vi "Reload.vi"(0 "reference in":refnum<class "LcWebView.lvclass">, 5 "Error In":errorcluster) -> (14 "reference out":refnum<class "LcWebView.lvclass">, 19 "Error Out":errorcluster)   [LabVIEW 2020, in "LcWebView.lvclass"]
uses:
  LcWebView.lvclass
  C:/Projects/WebView2/LcWebView/data/Microsoft.Web.WebView2.Core.dll
  data/Microsoft.Web.WebView2.Core.dll
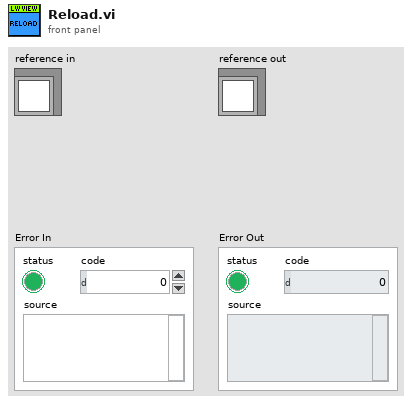
[diagram p1: front panel]
types:
  T1 = typedef "LcWebView.lvclass/ObjectAttributes.ctl" = cluster{"WebView Container":refnum<k24>, "CoreWebViewRef":refnum<k24>, "Status":i32, "Status Message":string, "User Data Folder":path, "DynamicEvents":T2, "BrowserProcessId":u32, "PlotMap":T3, "PlotType":T5}
  T2 = typedef "LcWebView.lvclass/WebViewDynamicEvents.ctl" = cluster{"Event Registration Ref":refnum<event-registration>, "Source event":refnum<user-event>}
  T3 = typedef "LcWebView.lvclass/PlotMap.ctl" = map{string, T4}
  T4 = typedef "LcWebView.lvclass/PlotRef.ctl" = cluster{"PlotType":T5, "PlotTemplate":string}
  T5 = typedef "LcWebView.lvclass/PlotType.ctl" = enum16{"bar", "line", "pie"}
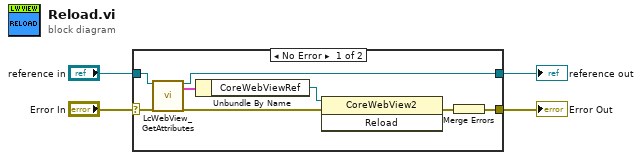
[diagram p0: block diagram]
diagram:
  n1 = case shown="No Error" "Error In" {
    selector: "Error In" -> [w12 w14]
    tunnel: [w9 w14] -> w3
    tunnel: [w10 w13] -> w1
    tunnel: "reference in" -> [w11 w13]
    frame No Error {
      n2 = call "LcWebView_GetAttributes.vi"("reference in"=w11, "error in (no error)"=w12) -> ("reference out"=w10:refnum<class "LcWebView.lvclass">, "Data"=w8:T1, "error out"=w6:errorcluster)  [unwired: 14 in, 1 out]
      n3 = Unbundle By Name(w8) -> ("CoreWebViewRef"=w7:refnum<k24>)
      n4 = invoke class="CoreWebView2" method="Reload"(reference=w7, error in=w6) -> (error out=w5:errorcluster)  [unwired: 1 in, 2 out]
      n5 = Merge Errors(w5) -> (w9:errorcluster)
    }
    frame Error {
    }
  }
  "Error Out" <- w3
  "reference out" <- w1
